vi "VI Server_M_ClmnListBox_SelectedCell_GET.vi"(4 "Selected Cell":T1, 7 "Label":string, 8 "error in":errorcluster, 10 "SingleInstance":bool=TRUE, 11 "VI Server.RefsCluster":T2) -> (0 "error out":errorcluster, 1 "Multicolumn Listbox.Ref":refnum<vi>, 2 "Cell.String":string, 3 "VI Server.RefsCluster.DUP":T2)   [LabVIEW 2020]
uses:
  VI Server_TypeDefs/VI Server_RefsCluster.ctl
  <vilib>/Utility/miscctls.llb/LVRowAndColumnTypeDef.ctl
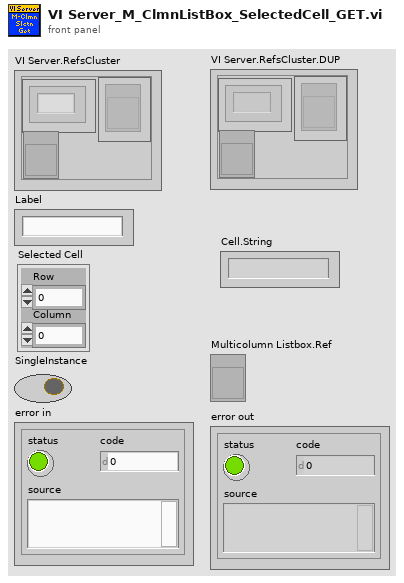
[diagram p1: front panel]
types:
  T1 = typedef "LVRowAndColumnTypeDef.ctl" = cluster{"Row":i32, "Column":i32}
  T2 = typedef "VI Server_RefsCluster.ctl" = cluster{"Labels":string[], "Refs":refnum<vi>[], "VI Ref":refnum<vi>}
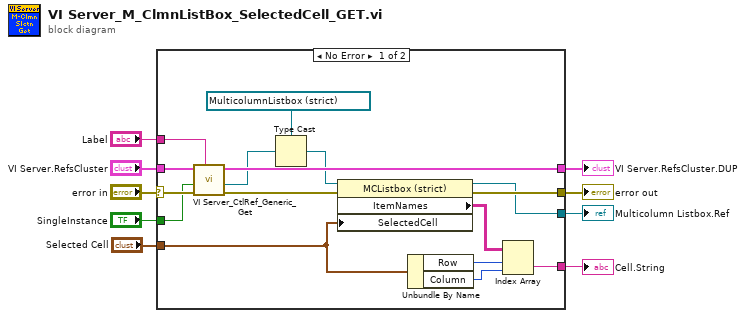
[diagram p0: block diagram]
diagram:
  n1 = case shown="No Error" "error in" {
    selector: "error in" -> [w25 w27]
    tunnel: [w16 w27] -> w8
    tunnel: "VI Server.RefsCluster" -> [w24 w26]
    tunnel: [w23 w26] -> w6
    tunnel: "Label" -> [w22 _]
    tunnel: "SingleInstance" -> [w18 _]
    tunnel: [w15 _] -> w3
    tunnel: "Selected Cell" -> [w13 _]
    tunnel: [w10 _] -> w1
    frame No Error {
      n2 = call "VI Server_CtlRef_Generic_Get.vi"("Control.Label"=w22, "error in"=w25, "SingleInstance"=w18, "VI Server.RefsCluster"=w24) -> ("error out"=w20:errorcluster, "Control.Ref.Generic"=w21:refnum<vi>, "VI Server.RefsCluster.DUP"=w23:T2)  [unwired: 5 in]
      n3 = Type Cast(type=refnum<vi> refnum ("Multicolumn Listbox"), x=w21) -> (*(type *) &x=w19:refnum<vi>)
      n4 = property class="MCListbox (strict)"(reference=w19, error in=w20, "SelectedCell"=w13) -> (reference out=w15:refnum<vi>, error out=w16:errorcluster, "ItemNames"=w14:string[][])
      n5 = Unbundle By Name(w13) -> ("Row"=w12:i32, "Column"=w11:i32)
      n6 = Index Array(array=w14, index (row)=w12, index (col)=w11) -> (element=w10:string)
    }
    frame Error {
    }
  }
  "VI Server.RefsCluster.DUP" <- w6
  "error out" <- w8
  "Multicolumn Listbox.Ref" <- w3
  "Cell.String" <- w1
